vi "Get next RUN.vi"(8 "error in (no error)":errorcluster, 11 "Monkey in":refnum<class "Monkey.lvclass">) -> (0 "error out":errorcluster, 2 "Current RUN":refnum<class "Run Instance.lvclass">, 3 "Monkey out":refnum<class "Monkey.lvclass">)   [LabVIEW 2020, in "Monkey.lvlib" / "Monkey.lvclass"]
doc: "Moves next run from the schedule to current RUN and returns its value"
uses:
  Monkey.lvclass
  Run Utilities/Run Instance/Run Instance.lvclass
  Run Utilities/Run Block/Run Block.lvclass
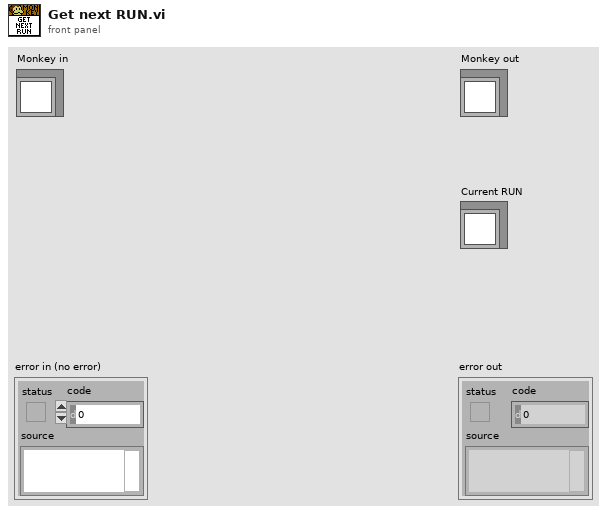
[diagram p1: front panel]
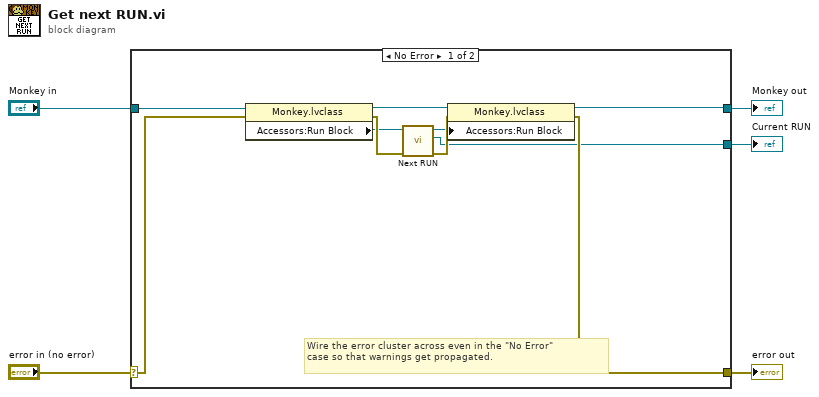
[diagram p0: block diagram]
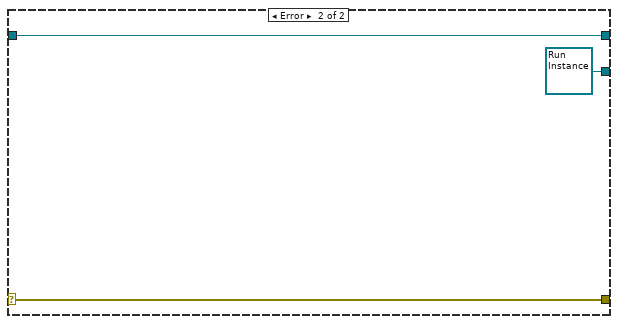
[diagram p2: hidden frame]
diagram:
  n1 = case shown="No Error" "error in (no error)" {
    selector: "error in (no error)" -> [w6 w18]
    tunnel: [w14 w18] -> w4
    tunnel: [w8 w17] -> w2
    tunnel: "Monkey in" -> [w10 w17]
    tunnel: [w7 refnum<class "Run Instance.lvclass"> refnum ("Current RUN")] -> w1
    frame No Error {
      # "Wire the error cluster across even in the \"No Error\"\ncase so that warnings get propagated."
      n2 = property class="Monkey.lvclass"(reference=w10, error in=w6) -> (reference out=w9:refnum<class "Monkey.lvclass">, error out=w13:errorcluster, "Accessors:Run Block"=w12:refnum<class "Run Block.lvclass">)
      n3 = call-dynamic "Next RUN.vi"("error in (no error)"=w13, "Run Block in"=w12) -> ("error out"=w15:errorcluster, "Current RUN"=w7:refnum<class "Run Instance.lvclass">, "Run Block out"=w11:refnum<class "Run Block.lvclass">)  [unwired: 7 in]
      n4 = property class="Monkey.lvclass"(reference=w9, error in=w15, "Accessors:Run Block"=w11) -> (reference out=w8:refnum<class "Monkey.lvclass">, error out=w14:errorcluster)
    }
    frame Error {
    }
  }
  "error out" <- w4
  "Monkey out" <- w2
  "Current RUN" <- w1
